vi "CMF - View Warmer.vi"(0 "Position Number":i8=1 min=0 max=40 step=1, 1 "Rack":u8=1 max=16, 2 "System":u8=1 min=1) -> ()   [LabVIEW 2021]
uses:
  Main Controls System v8.0/AutoAge Globals.vi
panel:
  in  "Update":bool
  in  "Exit":bool
  in  "Nominal Freq (fnom) Hz":dbl=10.0 min=0.0 max=400.0 step=1.0 format="%.6f"
  out "Initial Frequency (fo)":dbl format="%.4f"
  in  "Show All  Readings":bool=TRUE
  in  "Upper Range":dbl format="%.2f"
  in  "Lower Range":dbl format="%.2f"
  out "Number of Readings":i32
  in  "Unit for Deviation":u8(ring)=1 items=["ppm", "ppb"]
  out "Unit Start Date & Time":string
  in  "Units for Time":u8(ring)=2 items=["Seconds", "Minutes", "Hours", "Days"]
  out "Plot":cluster{dbl[], dbl[]}(graph)
  out "Max Delta":dbl format="%.3f"
  out "Elapsed Time":dbl format="%.2f"
  out "Serial Number":string
  # "Aging System - Warm -Up"
  # "Hz"
  # "Frequency\nChange\n( f t - f t0 )\n( fnom )"
  # "Time ( dt )"
  # "Range to View"
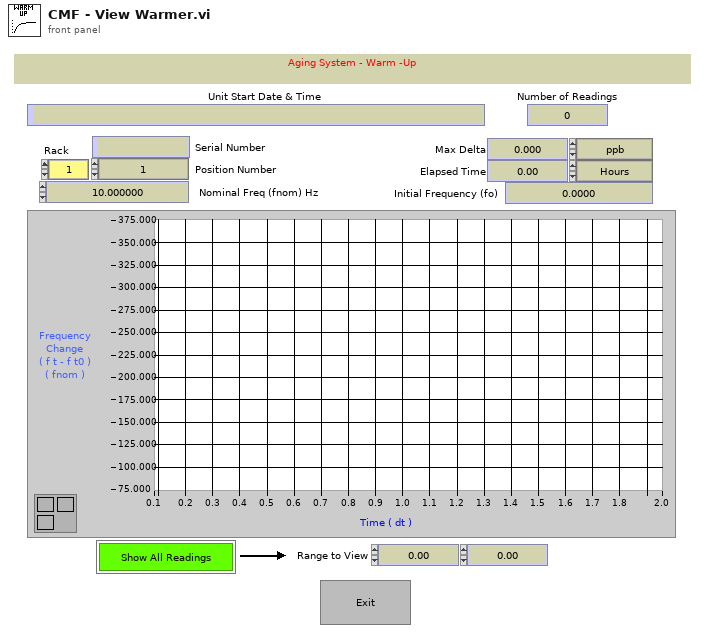
[diagram p1: front panel]
types:
  T1 = cluster{"Show All Readings":bool, "Upper Range":dbl, "Lower Range":dbl, "Time units":u8}
  T2 = cluster{"Time":dbl[], "Frequency(Hz)":dbl[], "Deltas(PPM)":dbl[]}
  T3 = cluster{"Serial Number":string, "Number of Readings":i32, "Initial Frequency (Hz)":dbl, "Unit Start Date & Time":string, "Nom Freq(MHz)":dbl}
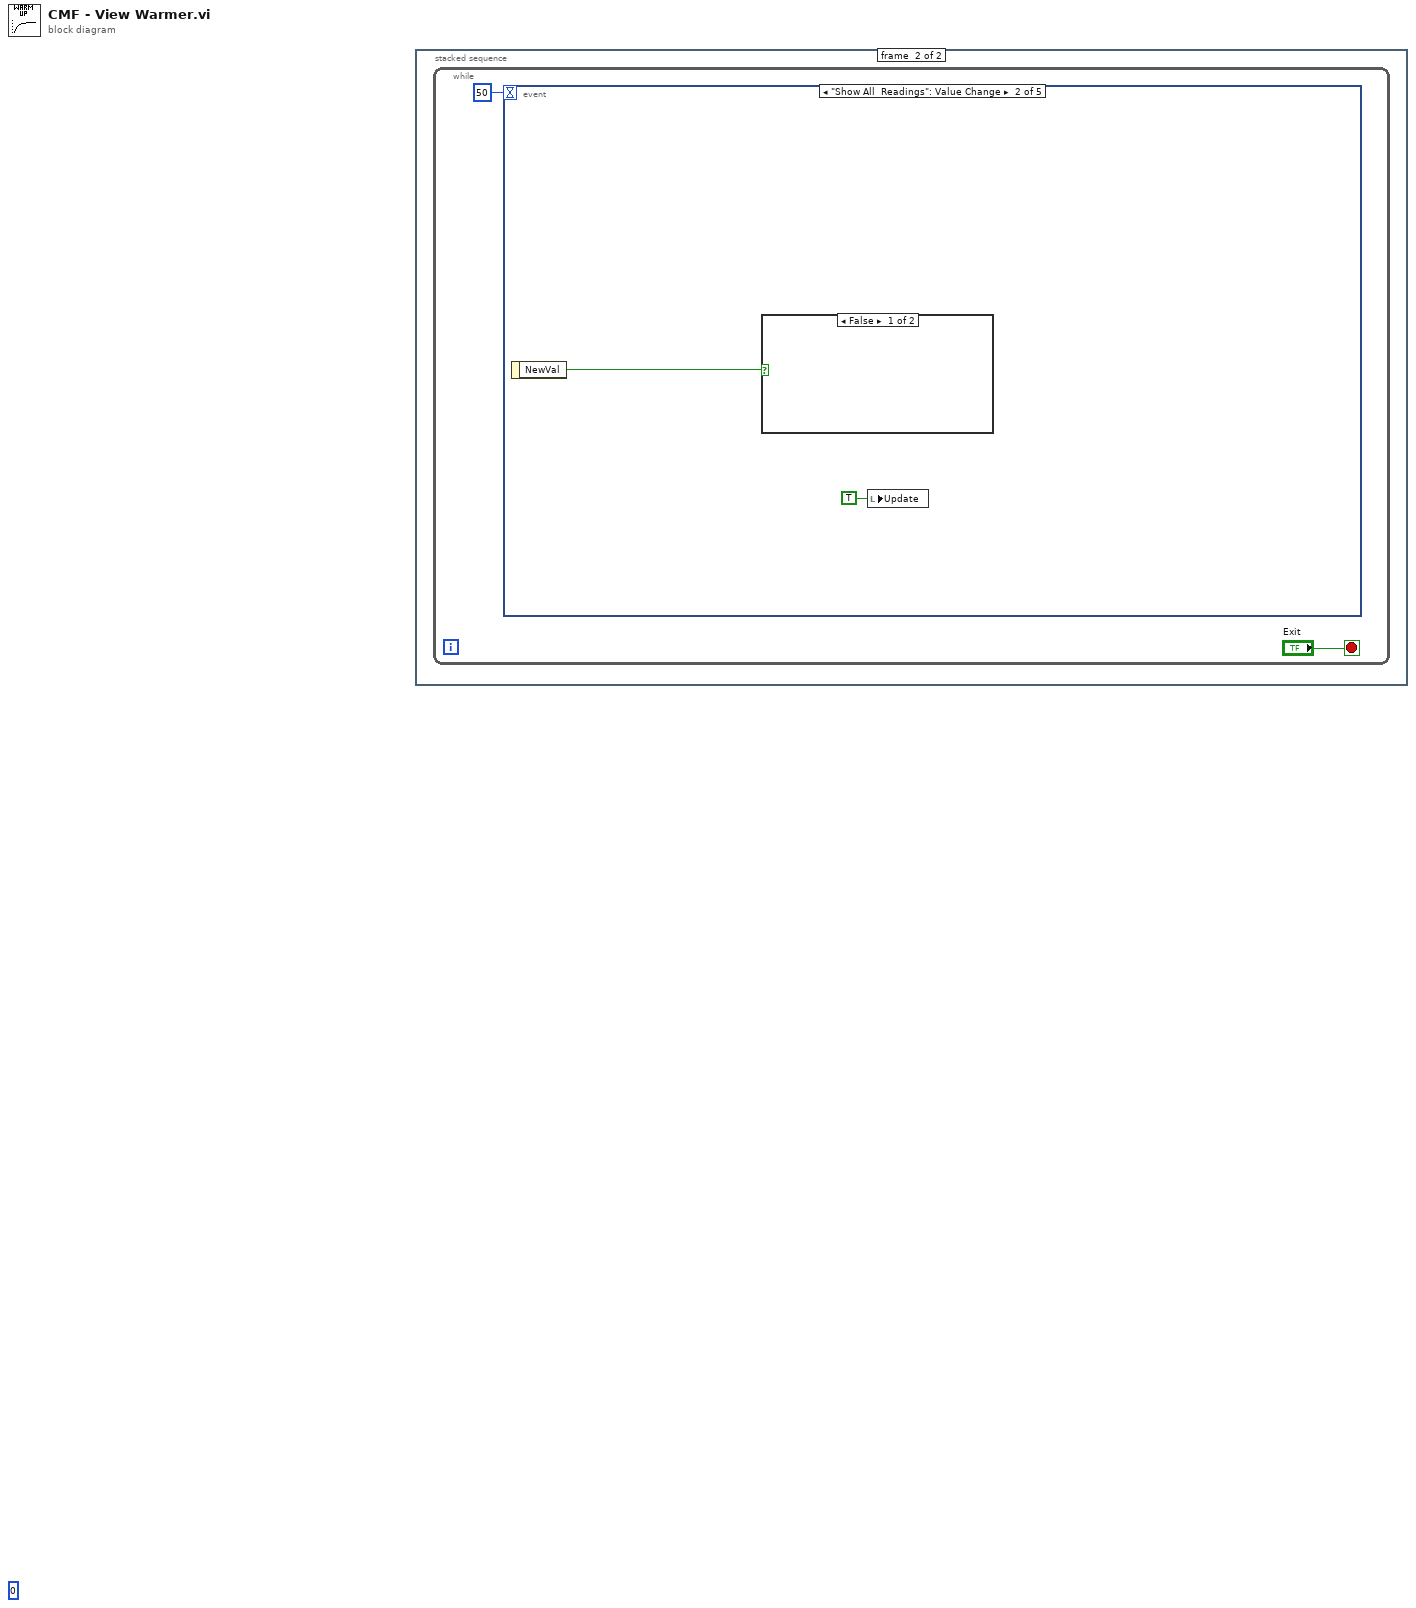
[diagram p0: block diagram]
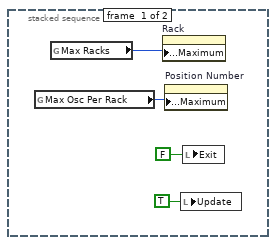
[diagram p2: hidden frame]
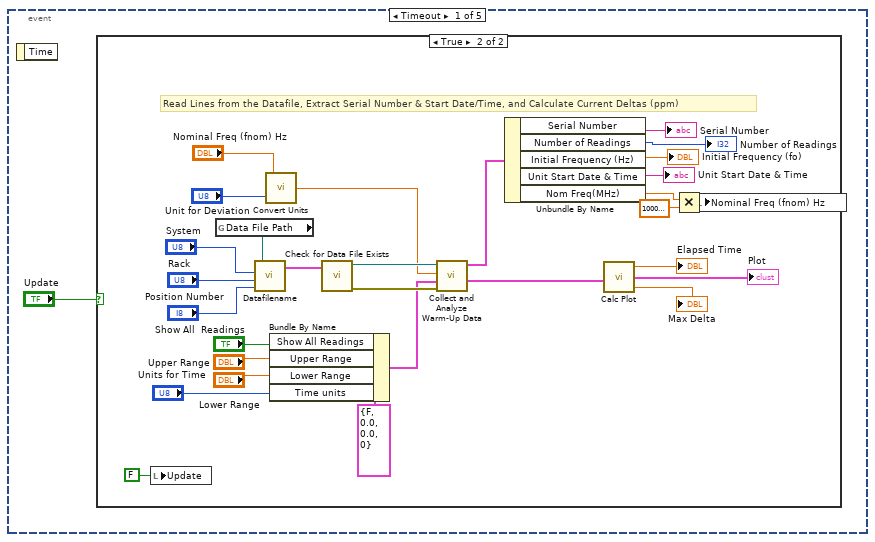
[diagram p3: hidden frame]
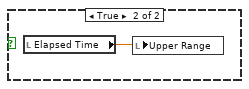
[diagram p5: hidden frame]
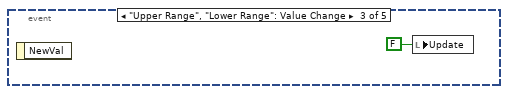
[diagram p6: hidden frame]
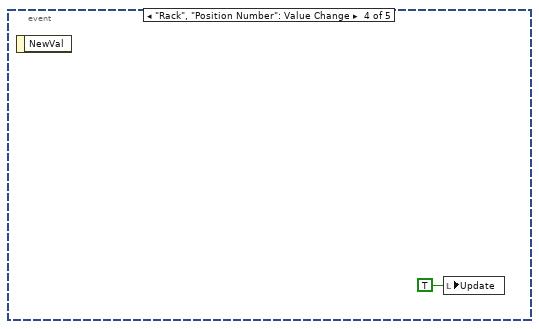
[diagram p7: hidden frame]
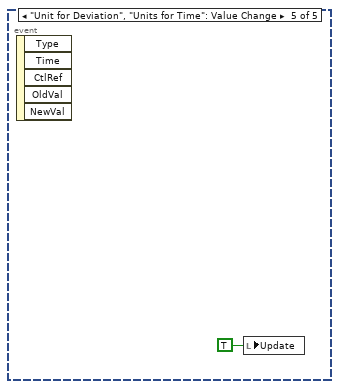
[diagram p8: hidden frame]
diagram:
  (unwired) u8 0 ("Units for Duration Under Test")
  n1 = stacked-sequence {
    frame #0 {
      n2 = global read "AutoAge Globals.vi" "Max Osc Per Rack"() -> (w2:u16)
      n3 = global read "AutoAge Globals.vi" "Max Racks"() -> (w3:u8)
      n4 = property on="Rack" class="DigNum (strict)"("Data Entry Limits:Maximum"=w3) -> ()  [unwired: 2 in, 2 out]
      n5 = property on="Position Number" class="DigNum (strict)"("Data Entry Limits:Maximum"=w2) -> ()  [unwired: 2 in, 2 out]
      n6 = local write "Update"(TRUE ("Update")) -> ()
      n7 = local write "Exit"(FALSE ("Exit")) -> ()
    }
    frame #1 {
      n8 = while {
        stop <- "Exit" stop-if-true
        n9 = event shown="[1] \"Show All  Readings\": Value Change" {
          selector: _ -> [_ _ _ _ _]
          dyn-events: _ -> [_ _ _ _ _]
          timeout: 50 -> [_ _ _ _ _]
          event Timeout {
            n10 = event-data() -> ()  [unwired: 1 in, 1 out]
            n11 = case shown="True" "Update" {
              frame False {
              }
              frame True {
                # "Read Lines from the Datafile, Extract Serial Number & Start Date/Time, and Calculate Current Deltas (ppm)"
                n12 = local write "Update"(FALSE ("Update")) -> ()
                n13 = global read "AutoAge Globals.vi" "Data File Path"() -> (w27:path)
                n14 = call "Datafilename.vi"("Position Number"="Position Number", "Rack"="Rack", "System"="System", "Data File Path"=w27) -> ("File Details"=w24:cluster{"Data Path":path, "Position Number":i8})
                n15 = call "Convert Units.vi"("Units for Duration Under Test"="Unit for Deviation", "Nominal Freq (fnom) Hz"="Nominal Freq (fnom) Hz") -> ("value"=w10:dbl)
                n16 = Bundle By Name(cluster=T1 {"Show All Readings"=FALSE, "Upper Range"=0.0, "Lower Range"=0.0, "Time units"=0} ("Range of Readings(time)"), "Show All Readings"="Show All  Readings", "Upper Range"="Upper Range", "Lower Range"="Lower Range", "Time units"="Units for Time") -> (w14:T1)
                n17 = call "Check for Data File Exists.vi"("File Details"=w24) -> ("error out"=w22:errorcluster, "refnum Out"=w28:refnum<file>)  [unwired: 1 in]
                n18 = call "Collect and Analyze Warm-Up Data.vi"("error in (no error)"=w22, "Range of Readings(time)"=w14, "Reference"=w10, "refnum"=w28) -> ("DataSets"=w21:T2, "Header"=w20:T3)  [unwired: 2 in, 1 out]
                n19 = Unbundle By Name(w20) -> ("Serial Number"=→"Serial Number":string, "Number of Readings"=→"Number of Readings":i32, "Initial Frequency (Hz)"=→"Initial Frequency (fo)":dbl, "Unit Start Date & Time"=→"Unit Start Date & Time":string, "Nom Freq(MHz)"=w17:dbl)
                n20 = call "Calc Plot.vi"("DataSets"=w21) -> ("Elapsed Time"=→"Elapsed Time":dbl, "Plot Data"=→"Plot":cluster{dbl[], dbl[]}, "Max Delta"=→"Max Delta":dbl)  [unwired: 1 in]
                n21 = Multiply(x=w17, y=1000000.0) -> (x*y=w36:dbl)
                n22 = local write "Nominal Freq (fnom) Hz"(w36) -> ()
              }
            }
          }
          event "Show All  Readings": Value Change {
            n23 = event-data() -> ("NewVal"=w37:bool)  [unwired: 1 in]
            n24 = case shown="False" w37 {
              frame False {
              }
              frame True {
                n25 = local read "Elapsed Time"() -> (w39:dbl)
                n26 = local write "Upper Range"(w39) -> ()
              }
            }
            n27 = local write "Update"(TRUE ("Update")) -> ()
          }
          event "Upper Range", "Lower Range": Value Change {
            n28 = event-data() -> ()  [unwired: 1 in, 1 out]
            n29 = local write "Update"(FALSE ("Update")) -> ()
          }
          event "Rack", "Position Number": Value Change {
            n30 = event-data() -> ()  [unwired: 1 in, 1 out]
            n31 = local write "Update"(TRUE ("Update")) -> ()
          }
          event "Unit for Deviation", "Units for Time": Value Change {
            n32 = event-data() -> ()  [unwired: 1 in, 5 out]
            n33 = local write "Update"(TRUE ("Update")) -> ()
          }
        }
      }
    }
  }
